vi "PH_StatusHandler.Status 2 String.vi"(1 "Status":T1 items=["no info", "off/false/out", "on/true/in", "Failure", "Alarm", "Status 1", "Status 2", "Status 3"]) -> (0 "Status as string":string)   [LabVIEW 2014, in "PH_StatusHandler.lvlib"]
doc: "This VI translates the state (I32) into a string."
uses:
  PH_StatusHandler.lvlib
  PH_StatusHandler.Status.ctl
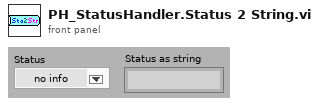
[diagram p1: front panel]
types:
  T1 = typedef "PH_StatusHandler.lvlib/PH_StatusHandler.Status.ctl" = i16
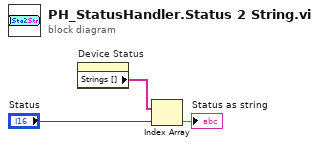
[diagram p0: block diagram]
diagram:
  n1 = property on="Device Status" class="Ring (strict)"() -> ("Strings []"=w1:string[])  [unwired: 2 in, 2 out]
  n2 = Index Array(array=w1, index="Status") -> (element=→"Status as string":string)
